vi "1553B_CMD_Get.vi"(7 "RT地址(默认：01111)":u16=15 format="%.0b", 9 "字长":u16=13, 11 "数据字数组":u16[](array[numeric])) -> (3 "1553B指令":string)   [LabVIEW 2012]
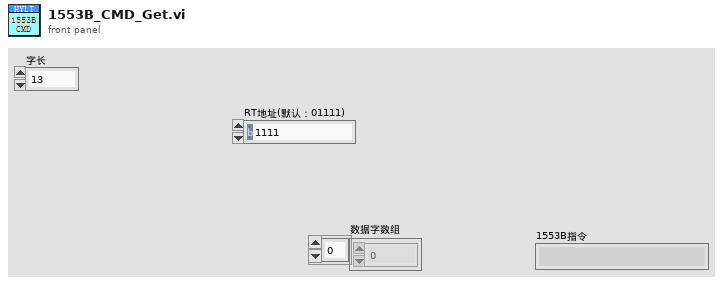
[diagram p1: front panel]
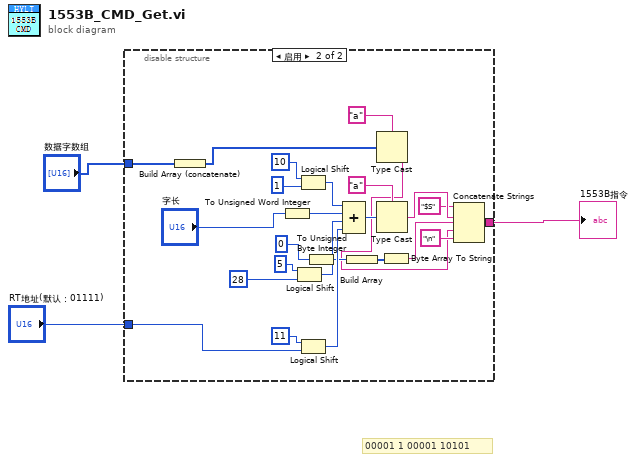
[diagram p0: block diagram]
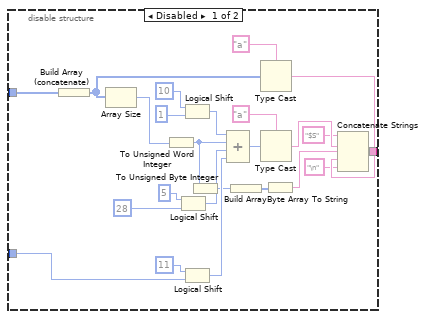
[diagram p2: hidden frame]
diagram:
  # "00001 1 00001 10101"
  n1 = disable-structure shown="启用" {
    disable-tunnel: "RT地址(默认：01111)" -> [w20 w29]
    disable-tunnel: [w11 w39] -> w2
    disable-tunnel: "数据字数组" -> [w10 w38]
    frame Disabled {
      n2 = Build Array (concatenate)(w10) -> (w9:u16[])
      n3 = Array Size(array=w9) -> (size(s)=w17:i32)
      n4 = To Unsigned Word Integer(number=w17) -> (unsigned 16bit integer=w8:u16)
      n5 = Logical Shift(y=i16 5, x=i16 28) -> (x << y=w23:i16)
      n6 = Logical Shift(y=i16 10, x=u16 1) -> (x << y=w24:u16)
      n7 = Logical Shift(y=i16 11, x=w20) -> (x << y=w19:u16)
      n8 = To Unsigned Byte Integer(number=w8) -> (unsigned 8bit integer=w6:u8)
      n9 = Compound Arithmetic op=ADD(w24, w8, w23, w19) -> (w18:u16)
      n10 = Build Array(w6) -> (w7:u8[])
      n11 = Type Cast(type="a" ("类型"), x=w9) -> (*(type *) &x=w15:string)
      n12 = Type Cast(type="a" ("类型"), x=w18) -> (*(type *) &x=w14:string)
      n13 = Byte Array To String(unsigned byte array=w7) -> (string=w5:string)
      n14 = Concatenate Strings("$S" ("字符串"), w14, w5, w15, "\n" ("字符串")) -> (w11:string)
    }
    frame Enabled {
      n15 = Build Array (concatenate)(w38) -> (w37:u16[])
      n16 = To Unsigned Word Integer(number="字长") -> (unsigned 16bit integer=w36:u16)
      n17 = Logical Shift(y=i16 5, x=i16 28) -> (x << y=w48:i16)
      n18 = Logical Shift(y=i16 10, x=u16 1) -> (x << y=w49:u16)
      n19 = Logical Shift(y=i16 11, x=w29) -> (x << y=w45:u16)
      n20 = To Unsigned Byte Integer(number=u8 0 ("数字")) -> (unsigned 8bit integer=w34:u8)
      n21 = Compound Arithmetic op=ADD(w49, w36, w48, w45) -> (w44:u16)
      n22 = Build Array(w34) -> (w35:u8[])
      n23 = Type Cast(type="a" ("类型"), x=w37) -> (*(type *) &x=w28:string)
      n24 = Type Cast(type="a" ("类型"), x=w44) -> (*(type *) &x=w42:string)
      n25 = Byte Array To String(unsigned byte array=w35) -> (string=w33:string)
      n26 = Concatenate Strings("$S" ("字符串"), w42, w33, w28, "\n" ("字符串")) -> (w39:string)
    }
  }
  "1553B指令" <- w2
